vi "Main.vi"() -> ()   [LabVIEW 2020]
panel:
  out "error out":errorcluster
  in  "停止":bool
  out "Image":T1(plugin-control)
  in  "Image Type":T2 items=["Grayscale (U8)", "Grayscale (I16)", "Grayscale (SGL)", "Complex (CSG)", "RGB (U32)", "HSL (U32)", "RGB (U64)", "Grayscale (U16)"]
  in  "File Path":path
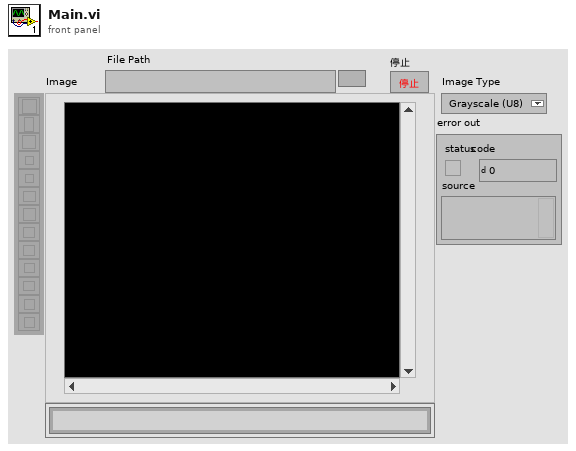
[diagram p1: front panel]
types:
  T1 = typedef "IMAQ Image.ctl" = refnum<image>
  T2 = typedef "Image Type" = u32
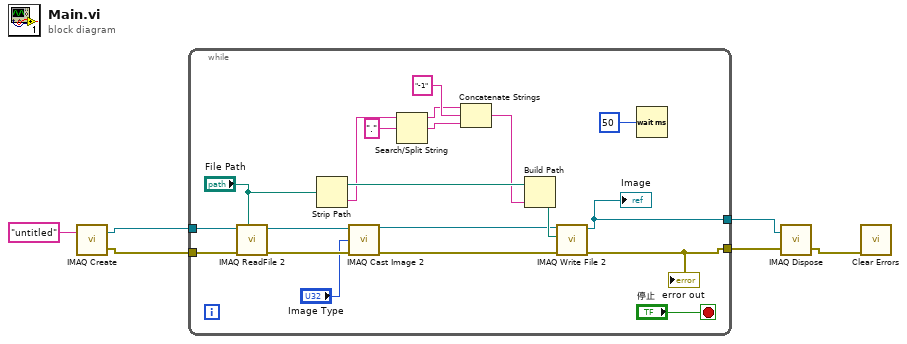
[diagram p0: block diagram]
diagram:
  n1 = call "IMAQ Create"("Image Name"="untitled") -> ("New Image"=w5:T1, "error out"=w4:errorcluster)  [unwired: 4 in]
  n2 = while {
    tunnel: w5 -> [w26]
    tunnel: w4 -> [w25]
    tunnel: [w7] -> w3
    tunnel: [w8] -> w2
    stop <- "停止" stop-if-true
    n3 = call "IMAQ ReadFile 2"("File Path"="File Path", "error in (no error)"=w25, "Image"=w26) -> ("error out"=w23:errorcluster, "Image Out"=w24:T1)  [unwired: 4 in, 3 out]
    n4 = Strip Path(path="File Path") -> (stripped path=w19:path, name=w15:string)
    n5 = call "IMAQ Cast Image 2"("Image Src"=w24, "Image Type"="Image Type", "error in (no error)"=w23) -> ("Image Dst Out"=w17:T1, "error out"=w22:errorcluster)  [unwired: 11 in]
    n6 = Search/Split String(string=w15, search string/char (-)="." ("搜索字符串/字符(-)")) -> (substring before match=w12:string, match + rest of string=w11:string)  [unwired: 1 in, 1 out]
    n7 = Concatenate Strings(w12, "-1", w11) -> (w10:string)
    n8 = Build Path(base path=w19, name or relative path=w10) -> (appended path=w18:path)
    n9 = call-poly "IMAQ Write File 2"("error in (no error)"=w22, "File Path"=w18, "Image"=w17) -> ("error out"=w7:errorcluster, "Image Out (duplicate)"=w8:T1)  [unwired: 7 in]
    "Image" <- w8
    "error out" <- w7
    n10 = Wait (ms)(milliseconds to wait=u32 50 ("等待时间（毫秒）")) -> ()  [unwired: 1 out]
  }
  n11 = call "IMAQ Dispose"("Image"=w2, "error in (no error)"=w3) -> ("error out"=w1:errorcluster)  [unwired: 4 in]
  n12 = call <vilib>:"Clear Errors.vi"("error in (no error)"=w1) -> ()  [unwired: 5 in, 2 out]
